vi "ExSubFullROI.vi"(2 "error in (no error)":errorcluster, 3 "Camera Handle":u32) -> (0 "error out":errorcluster, 1 "Camera Handle":u32)   [LabVIEW 2010]
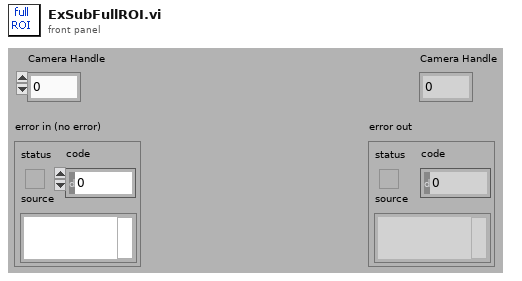
[diagram p1: front panel]
types:
  T1 = cluster{"X start":u32, "X end":u32, "X Binning/Grouping":u32, "Y start":u32, "Y end":u32, "Y Binning/Grouping":u32}
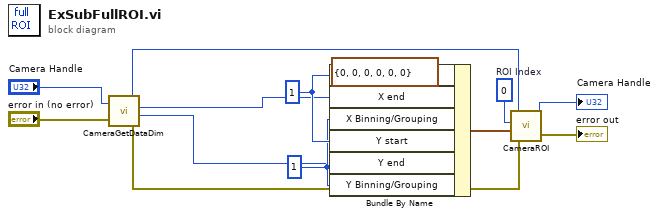
[diagram p0: block diagram]
diagram:
  w6 = u32 0  # ROI Index
  w4 = u32 1
  w5 = u32 1
  n1 = call <userlib>:"CameraGetDataDim.vi"("Camera Handle"="Camera Handle", "error in"="error in (no error)") -> ("Camera Handle"=w12:u32, "Xdim"=w2:u32, "Ydim"=w1:u32, "error out"=w10:errorcluster)
  n2 = Bundle By Name(cluster=T1 {"X start"=0, "X end"=0, "X Binning/Grouping"=0, "Y start"=0, "Y end"=0, "Y Binning/Grouping"=0} ("ROI Params"), "X start"=w5, "X end"=w2, "X Binning/Grouping"=w4, "Y start"=w5, "Y end"=w1, "Y Binning/Grouping"=w4) -> (w3:T1)
  n3 = call <userlib>:"CameraROI.vi"("error in"=w10, "ROI Params"=w3, "ROI Index"=w6, "Camera Handle"=w12) -> ("error out"=→"error out":errorcluster, "Camera Handle"=→"Camera Handle":u32)
